vi "Autonomous Independent.vi"() -> ()   [LabVIEW 2013]
doc: "This VI is called when autonomous begins, and will automatically be terminated when autonomous ends. You can carry out timed or sensor driven robot movement independently without needing to return to the caller."
uses:
  <vilib>/Rock Robotics/WPI/RobotDrive/WPI_RobotDriveArcadeDrive_Standard(NoSaturation).vi
  Robot Global Data.vi
panel:
  out "Current Movement, for debugging":T1 {"Y Joystick Value" scale=1.0..-1.0; "X Joystick Value" scale=-1.0..1.0}
  in  "Array of robot movements":T2(array[cluster]) {"Y Joystick Value" scale=1.0..-1.0; "X Joystick Value" scale=-1.0..1.0}
  # "Be sure to right-click and choose Data Operations>>Make Current Value default if you want to save the array values with the VI"
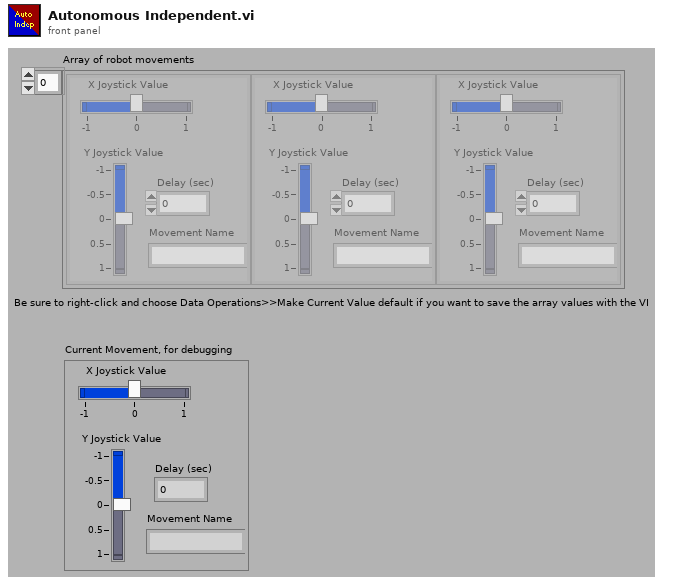
[diagram p1: front panel]
types:
  T1 = cluster{"X Joystick Value":dbl, "Y Joystick Value":dbl, "Delay (sec)":dbl, "Movement Name":string}
  T2 = cluster{"X Joystick Value":dbl, "Y Joystick Value":dbl, "Delay (sec)":dbl, "Movement Name":string}[]
  T3 = typedef "WPI_JoystickDevRef.ctl" = cluster{"Device":T4}
  T4 = typedef "WPI_JoystickDeviceEnum.ctl" = enum16{"USB 1", "USB 2", "USB 3", "USB 4", "Kinect 1", "Kinect 2"}
  T5 = cluster{"axis 1 (x)":dbl, "axis 2 (y)":dbl, "axis 3 (throttle)":dbl, "axis 4":dbl, "axis 5":dbl, "axis 6":dbl}
  T6 = typedef "WPI_MotorControlDeviceRef.ctl" = cluster{"DeviceStatus":errorcluster, "Type":enum16{"PWM", "CAN"}, "PWM":cluster{"Digital Module":T7, "PWM Channel":T8, "DeadBand":T9}, "CAN":cluster{"Device Number":u8, "Control Mode":T10, "Semaphore":T11, "Max Vout":dbl}, "Invert":bool, "TransformRef":T12, "InvTransformRef":T12}
  T7 = typedef "FPGA_TypedefDigitalModule.ctl" = enum16{"Digital Module 1", "Digital Module 2"}
  T8 = typedef "FPGA_DIOPWMChannel.ctl" = enum8{"PWM 1", "PWM 2", "PWM 3", "PWM 4", "PWM 5", "PWM 6", "PWM 7", "PWM 8", "PWM 9", "PWM 10", "Invalid"}
  T9 = typedef "WPI_PWMDeadband.ctl" = cluster{"Name":string, "maxPositivePwm":i32, "minPositivePwm":i32, "centerPwm":i32, "maxNegativePwm":i32, "minNegativePwm":i32, "angularRange":u16}
  T10 = typedef "WPI_CANJaguar_ControlMode.ctl" = enum8{"Percent VBus", "Current", "Speed", "Position", "Voltage"}
  T11 = typedef "Semaphore RefNum" = refnum<k1>
  T12 = typedef "WPI_PWMTransform_ConPane.ctl" = refnum<vi>
  T13 = typedef "WPI_RobotDriveDevRef.ctl" = cluster{"DevStatus":errorcluster, "Motors[]":T6[], "Square Inputs":bool, "Max Output":dbl, "Isochronous":bool}
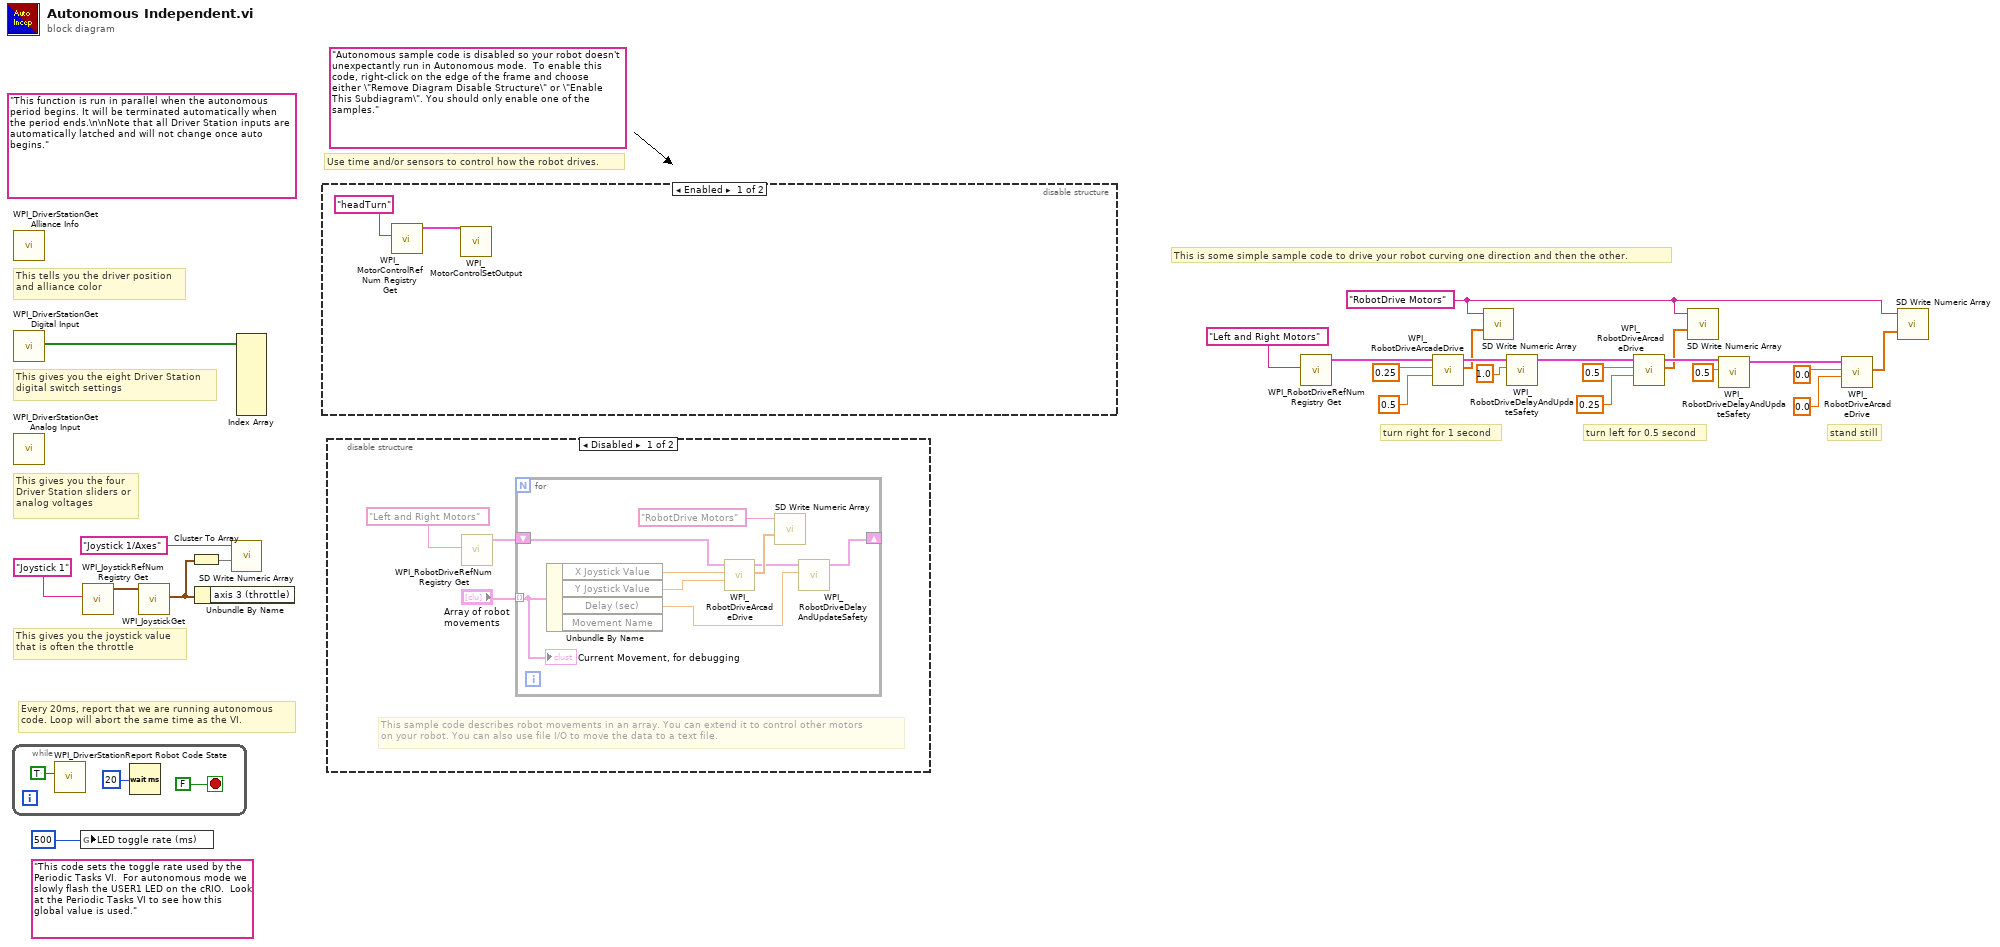
[diagram p0: block diagram]
diagram:
  w1 = "RobotDrive Motors" ("Name")
  (unwired) "This code sets the toggle rate used by the Periodic Tasks VI.  For autonomous mode we slowly flash the USER1 LED on the cRIO.  Look at the Periodic Tasks VI to see how this global value is used."
  (unwired) "Autonomous sample code is disabled so your robot doesn't unexpectantly run in Autonomous mode.  To enable this code, right-click on the edge of the frame and choose either \"Remove Diagram Disable Structure\" or \"Enable This Subdiagram\". You should only enable one of the samples."
  (unwired) "This function is run in parallel when the autonomous period begins. It will be terminated automatically when the period ends.\n\nNote that all Driver Station inputs are automatically latched and will not change once auto begins."
  # "This is some simple sample code to drive your robot curving one direction and then the other."
  # "stand still"
  # "turn left for 0.5 second"
  # "turn right for 1 second"
  # "Every 20ms, report that we are running autonomous\ncode. Loop will abort the same time as the VI."
  # "This gives you the joystick value\nthat is often the throttle"
  # "Use time and/or sensors to control how the robot drives."
  # "This tells you the driver position\nand alliance color"
  # "This gives you the eight Driver Station\ndigital switch settings"
  # "This gives you the four\nDriver Station sliders or\nanalog voltages"
  n1 = while {
    stop <- FALSE stop-if-true
    n2 = call <vilib>:"WPI_DriverStationReport Robot Code State.vi"("Autonomous"=TRUE) -> ()  [unwired: 10 in, 1 out]
    n3 = Wait (ms)(milliseconds to wait=u32 20) -> ()  [unwired: 1 out]
  }
  n4 = call <vilib>:"WPI_DriverStationGet Alliance Info.vi"() -> ()  [unwired: 12 out]
  n5 = call <vilib>:"WPI_DriverStationGet Digital Input.vi"() -> ("Driver Station Digital Input (1-8)"=w25:bool[])  [unwired: 11 out]
  n6 = call <vilib>:"WPI_DriverStationGet Analog Input.vi"() -> ()  [unwired: 12 out]
  n7 = global write "Robot Global Data.vi" "LED toggle rate (ms)"(u32 500 ("LED ms toggle rate")) -> ()
  n8 = call <vilib>:"WPI_JoystickRefNum Registry Get.vi"("refnum name"="Joystick 1") -> ("JoystickDevRef"=w23:T3)  [unwired: 1 in, 9 out]
  n9 = call <vilib>:"WPI_JoystickGet.vi"("JoystickDevRef"=w23) -> ("Axes"=w20:T5)  [unwired: 1 in, 5 out]
  n10 = Cluster To Array(cluster=w20) -> (array=w21:dbl[])
  n11 = Unbundle By Name(w20) -> ()  [unwired: 1 out]
  n12 = call <vilib>:"SD Write Numeric Array.vi"("Numeric Array"=w21, "Name"="Joystick 1/Axes") -> ()  [unwired: 8 in, 2 out]
  n13 = Index Array(array=w25) -> ()  [unwired: 8 in, 8 out]
  n14 = disable-structure shown="Enabled" {
    frame Enabled {
      n15 = call <vilib>:"WPI_MotorControlRefNum Registry Get.vi"("refnum name"="headTurn") -> ("MotorControlDevRef"=w29:T6)  [unwired: 9 in, 1 out]
      n16 = call <vilib>:"WPI_MotorControlSetOutput.vi"("MotorControlDevRef"=w29) -> ()  [unwired: 8 in, 3 out]
    }
    frame Disabled {
    }
  }
  n17 = disable-structure shown="Disabled" {
    frame Disabled {
      # "This sample code describes robot movements in an array. You can extend it to control other motors\non your robot. You can also use file I/O to move the data to a text file."
      n18 = call <vilib>:"WPI_RobotDriveRefNum Registry Get.vi"("refnum name"="Left and Right Motors") -> ("RobotDriveDevRef"=w32:T13)  [unwired: 1 in, 9 out]
      n19 = for {
        shift-right: [w38] -> _
        shift-left: w32 -> [w39]
        tunnel: "Array of robot movements" -> [w34] mode=indexing
        n20 = Unbundle By Name(w34) -> ("X Joystick Value"=w37:dbl, "Y Joystick Value"=w36:dbl, "Delay (sec)"=w35:dbl)  [unwired: 1 out]
        n21 = call-poly <vilib>:"WPI_RobotDriveArcadeDrive.vi"("Y axis value"=w36, "X axis value"=w37, "RobotDriveDevRef"=w39) -> ("Motor Values"=w41:dbl[], "RobotDriveDevRef"=w40:T13)  [unwired: 1 in, 6 out]
        n22 = call <vilib>:"SD Write Numeric Array.vi"("Numeric Array"=w41, "Name"="RobotDrive Motors") -> ()  [unwired: 8 in, 2 out]
        n23 = call <vilib>:"WPI_RobotDriveDelayAndUpdateSafety.vi"("Delay (s)"=w35, "RobotDriveDevRef"=w40) -> ("RobotDriveDevRef 2"=w38:T13)  [unwired: 8 in, 1 out]
        "Current Movement, for debugging" <- w34
      }
    }
    frame Enabled {
    }
  }
  n24 = call <vilib>:"WPI_RobotDriveRefNum Registry Get.vi"("refnum name"="Left and Right Motors") -> ("RobotDriveDevRef"=w5:T13)  [unwired: 1 in, 9 out]
  n25 = call-poly <vilib>:"WPI_RobotDriveArcadeDrive.vi"("Y axis value"=0.5 ("X axis value"), "X axis value"=0.25, "RobotDriveDevRef"=w5) -> ("Motor Values"=w4:dbl[], "RobotDriveDevRef"=w12:T13)  [unwired: 1 in, 6 out]
  n26 = call <vilib>:"SD Write Numeric Array.vi"("Numeric Array"=w4, "Name"=w1) -> ()  [unwired: 8 in, 2 out]
  n27 = call <vilib>:"WPI_RobotDriveDelayAndUpdateSafety.vi"("Delay (s)"=1.0, "RobotDriveDevRef"=w12) -> ("RobotDriveDevRef 2"=w11:T13)  [unwired: 8 in, 1 out]
  n28 = call-poly <vilib>:"WPI_RobotDriveArcadeDrive.vi"("Y axis value"=0.25 ("X axis value"), "X axis value"=0.5, "RobotDriveDevRef"=w11) -> ("Motor Values"=w3:dbl[], "RobotDriveDevRef"=w10:T13)  [unwired: 1 in, 6 out]
  n29 = call <vilib>:"SD Write Numeric Array.vi"("Numeric Array"=w3, "Name"=w1) -> ()  [unwired: 8 in, 2 out]
  n30 = call <vilib>:"WPI_RobotDriveDelayAndUpdateSafety.vi"("Delay (s)"=0.5, "RobotDriveDevRef"=w10) -> ("RobotDriveDevRef 2"=w9:T13)  [unwired: 8 in, 1 out]
  n31 = call-poly <vilib>:"WPI_RobotDriveArcadeDrive.vi"("Y axis value"=0.0 ("X axis value"), "X axis value"=0.0, "RobotDriveDevRef"=w9) -> ("Motor Values"=w2:dbl[])  [unwired: 1 in, 7 out]
  n32 = call <vilib>:"SD Write Numeric Array.vi"("Numeric Array"=w2, "Name"=w1) -> ()  [unwired: 8 in, 2 out]
